vi "Replace Outside Items.vi"(8 "error in":errorcluster, 9 "project:open":refnum<vi>, 10 "outside vis":string[](array[string]), 11 "destination directory":path) -> (0 "error out":errorcluster)   [LabVIEW 2021, in "Converter.lvlib"]
uses:
  Converter.lvlib
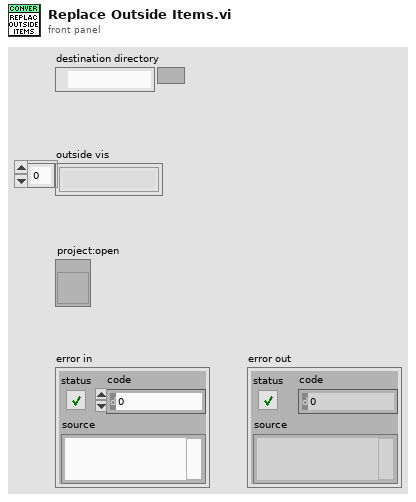
[diagram p1: front panel]
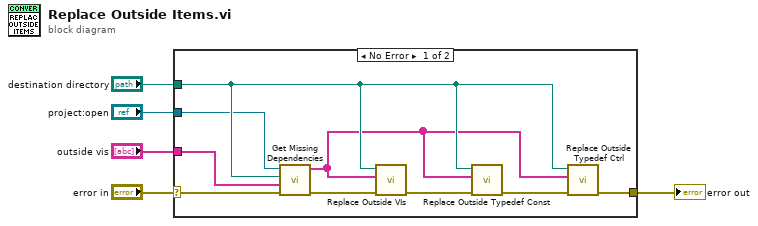
[diagram p0: block diagram]
diagram:
  n1 = case shown="No Error" "error in" {
    selector: "error in" -> [w6 w15]
    tunnel: "outside vis" -> [w14 _]
    tunnel: [w13 w15] -> w4
    tunnel: "destination directory" -> [w10 _]
    tunnel: "project:open" -> [w7 _]
    frame No Error {
      n2 = call "Get Missing Dependencies.vi"("error in"=w6, "outside vis in"=w14, "destination directory"=w10, "project in"=w7) -> ("error out"=w9:errorcluster, "outside vis out"=w8:string[])  [unwired: 6 in]
      n3 = call "Replace Outside VIs.vi"("error in"=w9, "non-library vi[]"=w8, "target directory"=w10) -> ("error out"=w11:errorcluster)  [unwired: 8 in]
      n4 = call "Replace Outside Typedef Const.vi"("error in"=w11, "non-library vi[]"=w8, "target directory"=w10) -> ("error out"=w12:errorcluster)  [unwired: 8 in]
      n5 = call "Replace Outside Typedef Ctrl.vi"("error in"=w12, "non-library vi[]"=w8, "target directory"=w10) -> ("error out"=w13:errorcluster)  [unwired: 8 in]
    }
    frame Error {
    }
  }
  "error out" <- w4
